vi "Load.vi"(8 "error in":errorcluster, 10 "Source":string, 11 "ConfiguratorJSON in":refnum<class "Config Hardcoded.lvclass">) -> (0 "error out":errorcluster, 3 "ConfiguratorJSON out":refnum<class "Config Hardcoded.lvclass">)   [LabVIEW 2024, in "PCAN.lvlib" / "Config Hardcoded.lvclass"]
uses:
  Config Hardcoded.lvclass
  Config Hardcoded.lvclass/Config Hardcoded.ctl
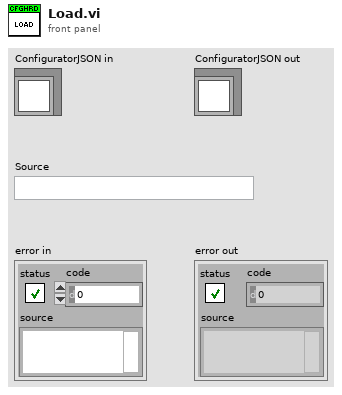
[diagram p1: front panel]
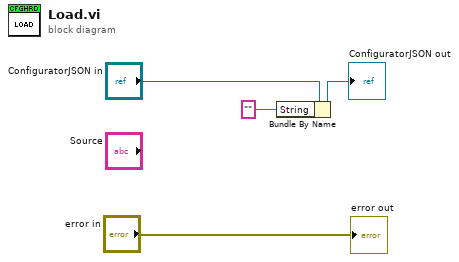
[diagram p0: block diagram]
diagram:
  n1 = Bundle By Name(cluster="ConfiguratorJSON in", "String"="") -> (→"ConfiguratorJSON out":refnum<class "Config Hardcoded.lvclass">)
  "error out" <- "error in"
